vi "_USB_CAN_DEBUG_LOG_OUT_.vi"(7 "Trans?":bool, 8 "id":u32, 9 "Info":string, 10 "Edata":i64[](array[numeric]), 11 "TIME":timestamp) -> ()   [LabVIEW 2011]
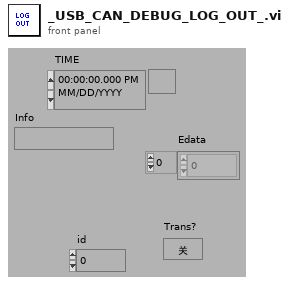
[diagram p1: front panel]
types:
  T1 = enum16{"open", "replace", "create", "open or create", "replace or create", "replace or create with confirmation"}
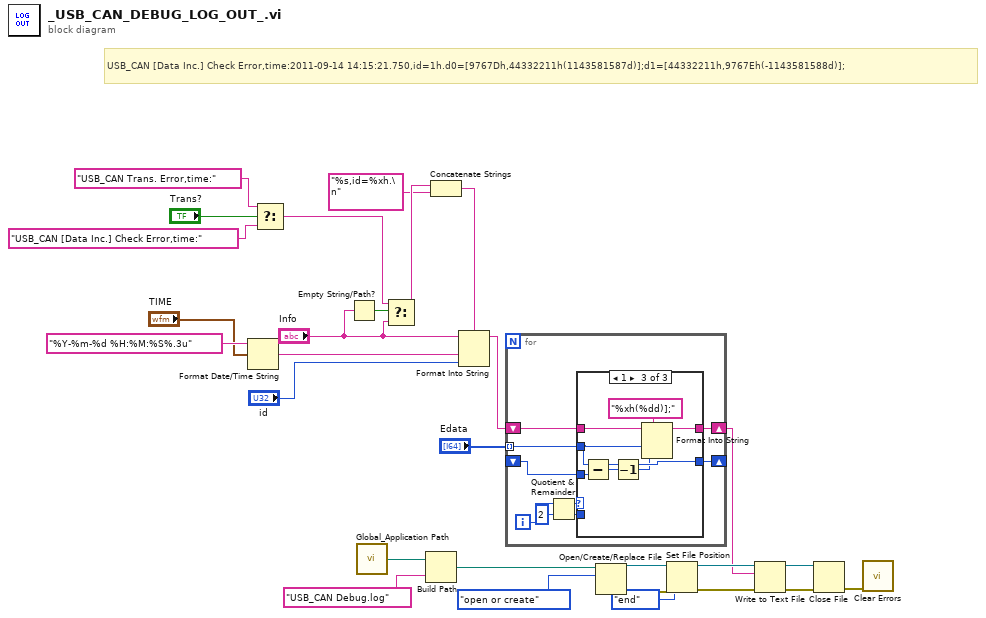
[diagram p0: block diagram]
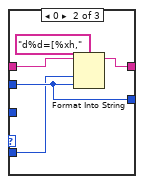
[diagram p3: hidden frame]
diagram:
  # "USB_CAN [Data Inc.] Check Error,time:2011-09-14 14:15:21.750,id=1h.d0=[9767Dh,44332211h(1143581587d)];d1=[44332211h,9767Eh(-1143581588d)];"
  n1 = Format Date/Time String(time format string (%c)="%Y-%m-%d %H:%M:%S%.3u" ("时间格式字符串(%c)"), seconds (now)="TIME") -> (date/time string=w26:string)  [unwired: 1 in]
  n2 = Select(t="USB_CAN Trans. Error,time:" ("格式字符串"), s="Trans?", f="USB_CAN [Data Inc.] Check Error,time:" ("格式字符串")) -> (s? t:f=w1:string)
  n3 = Empty String/Path?(string/path="Info") -> (empty?=w6:bool)
  n4 = call "Global_Application Path.vi"() -> ("程序路径"=w7:path)  [unwired: 1 in]
  n5 = Select(t=w1, s=w6, f="Info") -> (s? t:f=w4:string)
  n6 = Build Path(base path=w7, name or relative path="USB_CAN Debug.log" ("名称或相对路径")) -> (appended path=w23:path)
  n7 = Concatenate Strings(w4, "%s,id=%xh.\n" ("字符串")) -> (w2:string)
  n8 = Format Into String(format string=w2, initial string="Info", w26, "id") -> (resulting string=w13:string)  [unwired: 1 in, 1 out]
  n9 = for {
    tunnel: "Edata" -> [w32] mode=indexing
    shift-right: [w36] -> w12
    shift-left: w13 -> [w37]
    shift-right: [w31] -> _
    shift-left: _ -> [w30]
    i -> [w35]
    n10 = Quotient & Remainder(x=w35, y=2) -> (x-y*floor(x/y)=w33:i32, floor(x/y)=w29:i32)
    n11 = case shown="1" w33 {
      tunnel: w37 -> [w39 w44 w51]
      tunnel: [w39 w43 w50] -> w36
      tunnel: w32 -> [w38 w41 w47]
      tunnel: [w38 w41 w47] -> w31
      tunnel: w30 -> [_ _ w46]
      tunnel: w29 -> [_ w40 _]
      frame -1, Default {
      }
      frame 0 {
        n12 = Format Into String(format string="d%d=[%xh," ("格式字符串"), initial string=w44, w40, w41) -> (resulting string=w43:string)  [unwired: 1 in, 1 out]
      }
      frame 1 {
        n13 = Subtract(x=w47, y=w46) -> (x-y=w48:i64)
        n14 = Decrement(x=w48) -> (x-1=w45:i64)
        n15 = Format Into String(format string="%xh(%dd)];" ("格式字符串"), initial string=w51, w47, w45) -> (resulting string=w50:string)  [unwired: 1 in, 1 out]
      }
    }
  }
  n16 = Open/Create/Replace File(file path (use dialog)=w23, operation (0:open)=T1."open or create" ("操作(0:open)")) -> (refnum out=w21:refnum<file>, error out=w20:errorcluster)  [unwired: 4 in, 1 out]
  n17 = Set File Position(refnum=w21, from (0:start)=enum16{"start", "end", "current"}."end" ("自（0:起始）"), error in=w20) -> (refnum out=w18:refnum<file>, error out=w17:errorcluster)  [unwired: 1 in]
  n18 = Write to Text File(file (use dialog)=w18, text=w12, error in=w17) -> (refnum out=w15:refnum<file>, error out=w16:errorcluster)  [unwired: 1 in, 1 out]
  n19 = Close File(refnum=w15, error in=w16) -> (error out=w11:errorcluster)  [unwired: 1 out]
  n20 = call <vilib>:"Clear Errors.vi"("error in (no error)"=w11) -> ()  [unwired: 6 in, 1 out]
